vi "left2.vi"(7 "Parâmetros Ini 2":T2={"Gyro Port"=0, "Sensor - Left"=3, "Sensor - Right"=2, "     Color \nSensor Port"=1, "Kp Front"=0.5, "Motor speed"=-15, "Distance to street"=0.0, "Motor speed turns"=16, "Kp Curvas"=0.3} {"Kp Front" format="%.3f"; "Color \nSensor Port" items=["Port 1", "Port 2", "Port 3", "Port 4"]; "Sensor - Right" items=["Port 1", "Port 2", "Port 3", "Port 4"]; "Sensor - Left" items=["Port 1", "Port 2", "Port 3", "Port 4"]; "Gyro Port" items=["Port 1", "Port 2", "Port 3", "Port 4"]}, 9 "NXT/EV3":T1) -> (1 "NXT/EV3 2":T1)   [LabVIEW 2016]
uses:
  <vilib>/NXT/Subs/LVHSConnector.ctl
  <vilib>/NXT/LegoClasses/BrickReference/BrickReference.lvclass
  parametros.ctl
  <vilib>/NXT/Block Support/NXT_InputPort.ctl
  <vilib>/NXT/Block Support/NXT_OutputPort.ctl
  <vilib>/NXT/Dual Mode Library/Sensors/EV3_Gyro_Angle.vi
  <vilib>/NXT/NXTIO Xnodes/NXTIONodeSubVIs/NXTMoveMotors.vi
  <vilib>/NXT/NXTIO Xnodes/AddressXNode/NXTIOAddress.xnode
  <vilib>/NXT/NXTIO Xnodes/NXTIOXNode/NXTIO.xnode
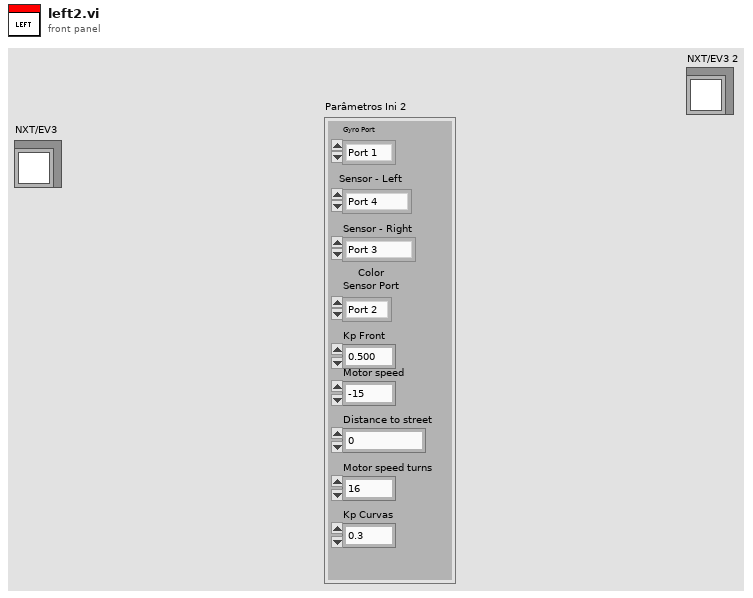
[diagram p1: front panel]
types:
  T1 = typedef "LVHSConnector.ctl" = refnum<class "BrickReference.lvclass">
  T2 = typedef "parametros.ctl" = cluster{"Gyro Port":T3, "Sensor - Left":T3, "Sensor - Right":T3, "     Color \nSensor Port":T3, "Kp Front":dbl, "Motor speed":i32, "Distance to street":dbl, "Motor speed turns":i32, "Kp Curvas":dbl}
  T3 = typedef "NXT_InputPort.ctl" = u32
  T4 = typedef "NXT_OutputPort.ctl" = u8
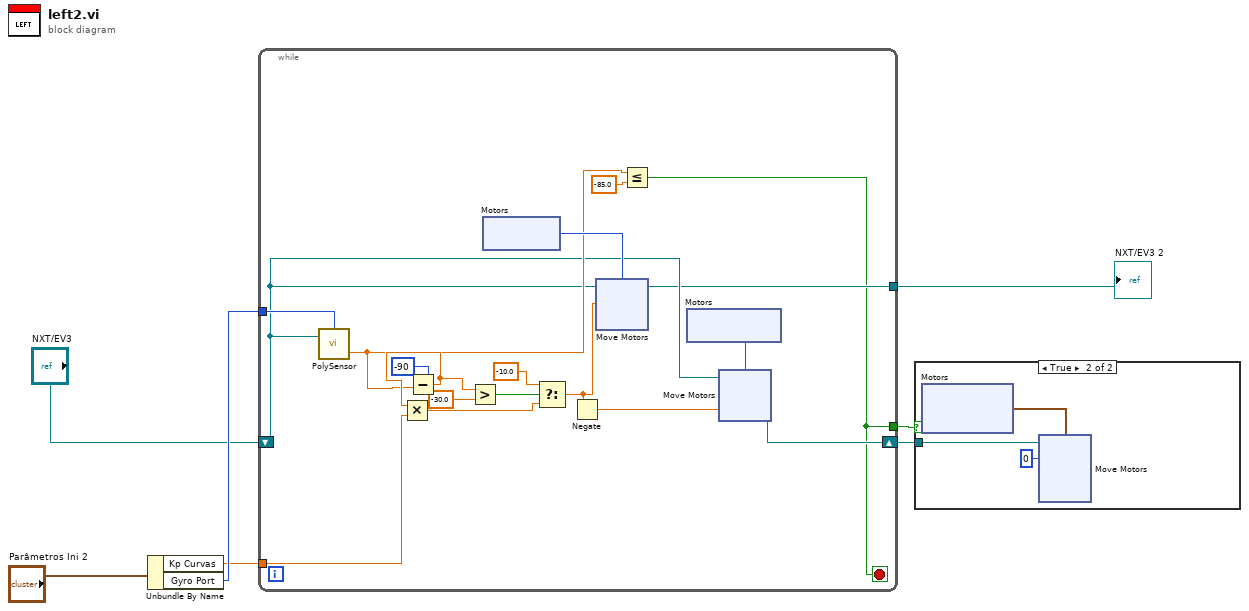
[diagram p0: block diagram]
diagram:
  n1 = Unbundle By Name("Parâmetros Ini 2") -> ("Kp Curvas"=w5:dbl, "Gyro Port"=w7:T3)
  n2 = while {
    tunnel: w7 -> [w25]
    tunnel: w5 -> [w24]
    tunnel: [w9] -> w2
    shift-right: [w10] -> w3
    shift-left: "NXT/EV3" -> [w11]
    tunnel: [w8] -> w1
    stop <- w8 stop-if-true
    n3 = call-poly <vilib>:"PolySensor.vi"("NXT/EV3"=w11, "Port (Port 1)"=w25) -> ("Degrees"=w14:sgl)  [unwired: 1 in, 1 out]
    n4 = Subtract(x=-90, y=w14) -> (x-y=w17:sgl)
    n5 = Multiply(x=w17, y=w24) -> (x*y=w15:dbl)
    n6 = Greater?(x=w17, y=sgl -30.0) -> (0:w21:bool)
    n7 = xnode "Motors"() -> ("Motor"=w20:T4)
    n8 = Select(t=sgl -10.0, s=w21, f=w15) -> (s? t:f=w12:dbl)
    n9 = Negate(x=w12) -> (-x=w13:dbl)
    n10 = xnode "Move Motors"("Power/Speed 1"=w12, "Motors"=w20, "NXT/EV3"=w11) -> ("NXT/EV3"=w9:T1)
    n11 = Less Or Equal?(x=w14, y=sgl -85.0) -> (x <= y?=w8:bool)
    n12 = xnode "Motors"() -> ("Motor"=w19:T4)
    n13 = xnode "Move Motors"("Power/Speed 1"=w13, "Motors"=w19, "NXT/EV3"=w11) -> ("NXT/EV3"=w10:T1)
  }
  "NXT/EV3 2" <- w2
  n14 = case shown="True" w1 {
    tunnel: w3 -> [_ w43]
    frame False {
    }
    frame True {
      w42 = i8 0 ("Power/Speed 1")
      n15 = xnode "Motors"() -> ("Motor"=w44:cluster{"Port":T4, "Port":T4})
      n16 = xnode "Move Motors"("Power/Speed 2"=w42, "Power/Speed 1"=w42, "Motors"=w44, "NXT/EV3"=w43) -> ()  [unwired: 1 out]
    }
  }
